vi "RGB to HSV and range.vi"(0 "Image Pixels (RGB)":u8[][][](array[numeric]), 2 "Hue Range":cluster{"Lower":u8, "Upper":u8}, 3 "Sat Range":cluster{"Lower":u8, "Upper":u8}) -> (7 "Threshholded Pixels":u8[][](array[numeric]))   [LabVIEW 2017]
doc: "Converts RGB values from a 3x320x240 pixel array to HSV values. Then determines if the hue and sat values are within a hue and saturation range and outputs a binary 320x240 array."
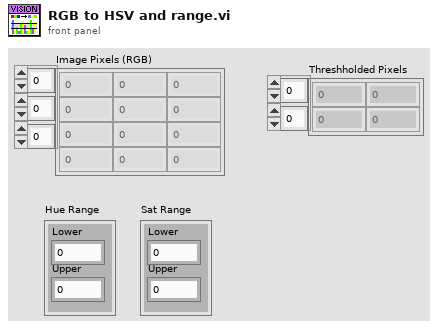
[diagram p1: front panel]
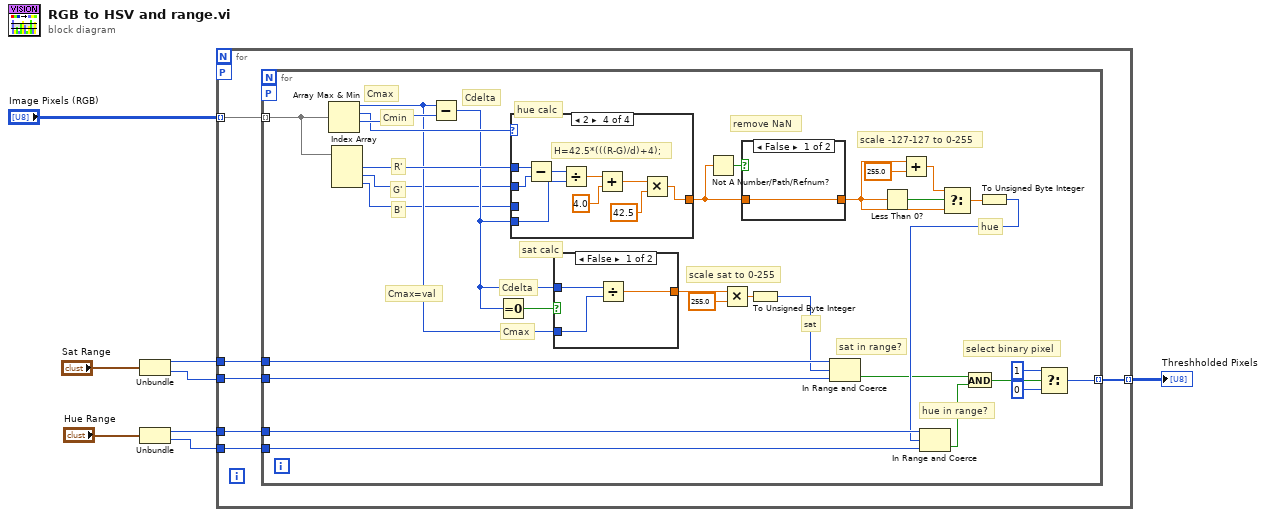
[diagram p0: block diagram]
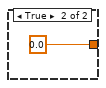
[diagram p2: hidden frame]
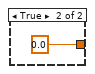
[diagram p3: hidden frame]
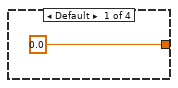
[diagram p4: hidden frame]
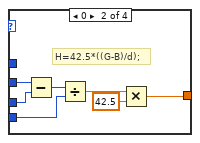
[diagram p5: hidden frame]
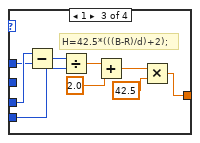
[diagram p6: hidden frame]
diagram:
  n1 = Unbundle("Sat Range") -> ("Lower"=w2:u8, "Upper"=w1:u8)
  n2 = Unbundle("Hue Range") -> ("Lower"=w5:u8, "Upper"=w4:u8)
  n3 = for {
    tunnel: "Image Pixels (RGB)" -> [w10] mode=indexing
    tunnel: w2 -> [w14]
    tunnel: w1 -> [w13]
    tunnel: w5 -> [w12]
    tunnel: w4 -> [w11]
    tunnel: [w9] -> w7 mode=indexing
    workers-P: _ -> [_]
    n4 = for {
      tunnel: w10 -> [w21] mode=indexing
      tunnel: w14 -> [w29]
      tunnel: w13 -> [w27]
      tunnel: w12 -> [w26]
      tunnel: w11 -> [w25]
      tunnel: [w17] -> w9 mode=indexing
      workers-P: _ -> [_]
      # "Cmin"
      # "Cmax"
      # "scale sat to 0-255"
      # "select binary pixel"
      # "hue in range?"
      # "sat in range?"
      # "sat"
      # "hue"
      # "Cmax=val"
      # "Cmax"
      # "Cdelta"
      # "sat calc"
      # "remove NaN"
      # "scale -127-127 to 0-255"
      # "hue calc"
      # "Cdelta"
      # "B'"
      # "G'"
      # "R'"
      n5 = Array Max & Min(array=w21) -> (max value=w32:u8, max index (indices)=w43:i32, min value=w45:u8)  [unwired: 1 out]
      n6 = Index Array(array=w21) -> (element #1=w44:u8, element #2=w20:u8, element #3=w19:u8)  [unwired: 3 in]
      n7 = Subtract(x=w32, y=w45) -> (x-y=w33:u8)
      n8 = Equal To 0?(x=w33) -> (x = 0?=w34:bool)
      n9 = case shown="2" w43 {
        tunnel: [0.0 w53 w62 w69] -> w36
        tunnel: w33 -> [_ w56 w67 w74]
        tunnel: w44 -> [_ _ w60 w77]
        tunnel: w20 -> [_ w59 _ w76]
        tunnel: w19 -> [_ w58 w61 _]
        frame Default {
        }
        frame 0 {
          # "H=42.5*((G-B)/d);"
          n10 = Subtract(x=w59, y=w58) -> (x-y=w57:u8)
          n11 = Divide(x=w57, y=w56) -> (x/y=w55:dbl)
          n12 = Multiply(x=w55, y=42.5) -> (x*y=w53:dbl)
        }
        frame 1 {
          # "H=42.5*(((B-R)/d)+2);"
          n13 = Subtract(x=w61, y=w60) -> (x-y=w68:u8)
          n14 = Divide(x=w68, y=w67) -> (x/y=w66:dbl)
          n15 = Add(x=w66, y=2.0) -> (x+y=w64:dbl)
          n16 = Multiply(x=w64, y=42.5) -> (x*y=w62:dbl)
        }
        frame 2 {
          # "H=42.5*(((R-G)/d)+4);"
          n17 = Subtract(x=w77, y=w76) -> (x-y=w75:u8)
          n18 = Divide(x=w75, y=w74) -> (x/y=w73:dbl)
          n19 = Add(x=w73, y=4.0) -> (x+y=w71:dbl)
          n20 = Multiply(x=w71, y=42.5) -> (x*y=w69:dbl)
        }
      }
      n21 = case shown="False" w34 {
        tunnel: [w46 0.0] -> w35
        tunnel: w32 -> [w47 _]
        tunnel: w33 -> [w48 _]
        frame False {
          n22 = Divide(x=w48, y=w47) -> (x/y=w46:dbl)
        }
        frame True {
        }
      }
      n23 = Not A Number/Path/Refnum?(number/path/refnum=w36) -> (NaN/Path/Refnum?=w39:bool)
      n24 = Multiply(x=w35, y=255.0) -> (x*y=w31:dbl)
      n25 = case shown="False" w39 {
        tunnel: w36 -> [w50 _]
        tunnel: [w50 0.0] -> w38
        frame False {
        }
        frame True {
        }
      }
      n26 = To Unsigned Byte Integer(number=w31) -> (unsigned 8bit integer=w28:u8)
      n27 = In Range and Coerce(upper limit=w29, x=w28, lower limit=w27) -> (In Range?=w23:bool)  [unwired: 1 out]
      n28 = Less Than 0?(x=w38) -> (x < 0?=w42:bool)
      n29 = Add(x=w38, y=255.0) -> (x+y=w40:dbl)
      n30 = Select(t=w40, s=w42, f=w38) -> (s? t:f=w37:dbl)
      n31 = To Unsigned Byte Integer(number=w37) -> (unsigned 8bit integer=w24:u8)
      n32 = In Range and Coerce(upper limit=w26, x=w24, lower limit=w25) -> (In Range?=w22:bool)  [unwired: 1 out]
      n33 = And(x=w23, y=w22) -> (x .and. y?=w18:bool)
      n34 = Select(t=u8 1, s=w18, f=u8 0) -> (s? t:f=w17:u8)
    }
  }
  "Threshholded Pixels" <- w7
